vi "Base64.vi"(1 "Switch":enum16{"Base 64 Encode", "Base 64 Decode"}(ring), 2 "Input String":string, 4 "OutputFileStructure":bool) -> (6 "Output String":string)   [LabVIEW 2019, in "HTTP Server.lvlib"]
uses:
  HTTP Server.lvlib
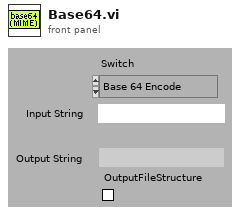
[diagram p1: front panel]
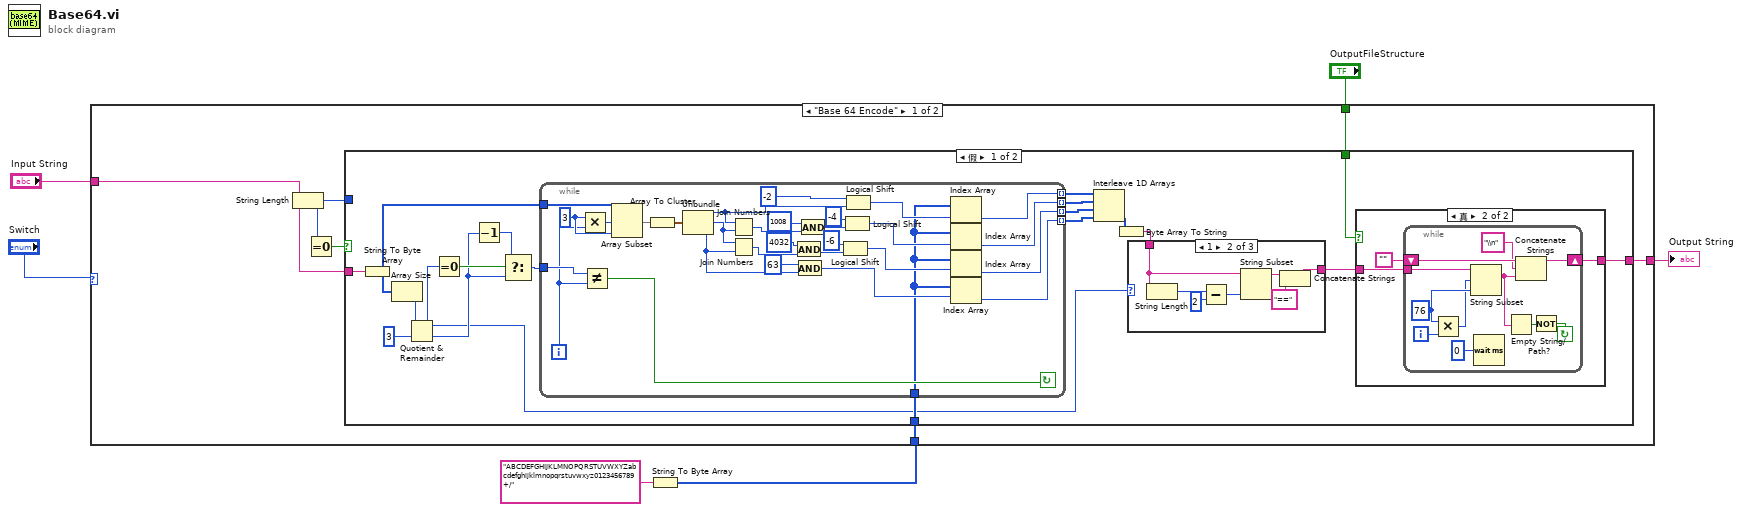
[diagram p0: block diagram]
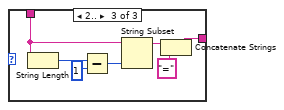
[diagram p3: hidden frame]
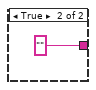
[diagram p5: hidden frame]
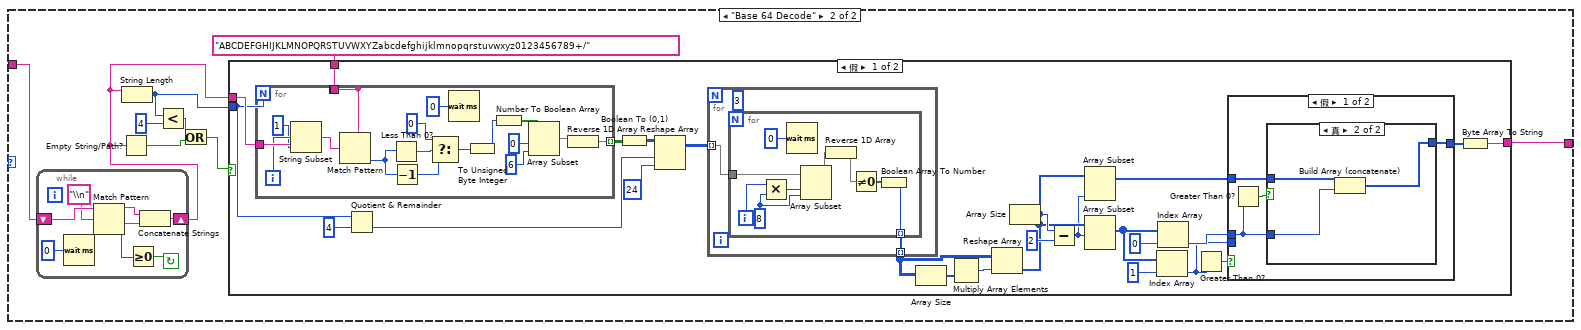
[diagram p6: hidden frame]
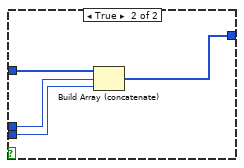
[diagram p8: hidden frame]
diagram:
  n1 = String To Byte Array(string="ABCDEFGHIJKLMNOPQRSTUVWXYZabcdefghijklmnopqrstuvwxyz0123456789+/") -> (unsigned byte array=w1:u8[])
  n2 = case shown="\"Base 64 Encode\"" "Switch" {
    tunnel: "Input String" -> [w12 w94]
    tunnel: "OutputFileStructure" -> [w11 _]
    tunnel: [w10 w98] -> w3
    tunnel: w1 -> [w7 _]
    frame "Base 64 Encode" {
      n3 = String Length(string=w12) -> (length=w8:i32)
      n4 = Equal To 0?(x=w8) -> (x = 0?=w9:bool)
      n5 = case shown="假" w9 {
        tunnel: [w31 ""] -> w10
        tunnel: w11 -> [w30 _]
        tunnel: w12 -> [w22 _]
        tunnel: w8 -> [_ _]
        tunnel: w7 -> [w24 _]
        frame False {
          n6 = String To Byte Array(string=w22) -> (unsigned byte array=w21:u8[])
          n7 = Array Size(array=w21) -> (size(s)=w25:i32)
          n8 = Quotient & Remainder(x=w25, y=3) -> (x-y*floor(x/y)=w14:i32, floor(x/y)=w28:i32)
          n9 = Equal To 0?(x=w14) -> (x = 0?=w29:bool)
          n10 = Decrement(x=w28) -> (x-1=w27:i32)
          n11 = Select(t=w27, s=w29, f=w28) -> (s? t:f=w23:i32)
          n12 = while {
            tunnel: [w32] -> w17 mode=indexing
            tunnel: [w33] -> w18 mode=indexing
            tunnel: [w34] -> w19 mode=indexing
            tunnel: [w35] -> w20 mode=indexing
            tunnel: w23 -> [w56]
            tunnel: w24 -> [w36]
            tunnel: w21 -> [w61]
            i -> [w55]
            stop <- w54 continue-if-true
            w59 = 3 ("x")
            n13 = Multiply(x=w59, y=w55) -> (x*y=w60:i32)
            n14 = Not Equal?(x=w56, y=w55) -> (x != y?=w54:bool)
            n15 = Array Subset(array=w61, index=w60, length=w59) -> (w57:u8[])
            n16 = Array To Cluster(array=w57) -> (cluster=w58:cluster{"[0]":u8, "[1]":u8, "[2]":u8})
            n17 = Unbundle(w58) -> ("[0]"=w43:u8, "[1]"=w48:u8, "[2]"=w42:u8)
            n18 = Join Numbers(hi=w43, lo=w48) -> ((hi.lo)=w52:u16)
            n19 = Join Numbers(hi=w48, lo=w42) -> ((hi.lo)=w47:u16)
            n20 = And(x=u16 4032, y=w47) -> (x .and. y?=w45:u16)
            n21 = And(x=u8 63, y=w42) -> (x .and. y?=w37:u8)
            n22 = And(x=u16 1008, y=w52) -> (x .and. y?=w50:u16)
            n23 = Logical Shift(y=i8 -6, x=w45) -> (x << y=w38:u16)
            n24 = Logical Shift(y=i8 -4, x=w50) -> (x << y=w39:u16)
            n25 = Logical Shift(y=i8 -2, x=w43) -> (x << y=w40:u8)
            n26 = Index Array(array=w36, index=w40) -> (element=w35:u8)
            n27 = Index Array(array=w36, index=w39) -> (element=w34:u8)
            n28 = Index Array(array=w36, index=w38) -> (element=w33:u8)
            n29 = Index Array(array=w36, index=w37) -> (element=w32:u8)
          }
          n30 = Interleave 1D Arrays(w20, w19, w18, w17) -> (w16:u8[])
          n31 = Byte Array To String(unsigned byte array=w16) -> (string=w15:string)
          n32 = case shown="1" w14 {
            tunnel: w15 -> [w62 w64 w71]
            tunnel: [w62 w63 w70] -> w13
            frame ..0 {
            }
            frame 1 {
              n33 = String Length(string=w64) -> (length=w68:i32)
              n34 = Subtract(x=w68, y=i16 2) -> (x-y=w67:i32)
              n35 = String Subset(string=w64, length (rest)=w67) -> (substring=w65:string)  [unwired: 1 out]
              n36 = Concatenate Strings(w65, "==") -> (w63:string)
            }
            frame 2.. {
              n37 = String Length(string=w71) -> (length=w75:i32)
              n38 = Subtract(x=w75, y=i16 1) -> (x-y=w74:i32)
              n39 = String Subset(string=w71, length (rest)=w74) -> (substring=w72:string)  [unwired: 1 out]
              n40 = Concatenate Strings(w72, "=") -> (w70:string)
            }
          }
          n41 = case shown="真" w30 {
            tunnel: [w77 w79] -> w31
            tunnel: w13 -> [w77 w78]
            frame False {
            }
            frame True {
              n42 = while {
                shift-left: "" -> [w88]
                shift-right: [w87] -> w79
                tunnel: w78 -> [w81]
                i -> [w91]
                stop <- w84 continue-if-true
                w90 = 76 ("length")
                n43 = Multiply(x=w90, y=w91) -> (x*y=w89:i32)
                n44 = String Subset(string=w81, offset (0)=w89, length (rest)=w90) -> (substring=w83:string)
                n45 = Wait (ms)(milliseconds to wait=u32 0) -> ()  [unwired: 1 out]
                n46 = Empty String/Path?(string/path=w83) -> (empty?=w85:bool)
                n47 = Concatenate Strings(w88, "\\n", w83) -> (w87:string)
                n48 = Not(x=w85) -> (.not. x?=w84:bool)
              }
            }
          }
        }
        frame True {
        }
      }
    }
    frame "Base 64 Decode" {
      n49 = while {
        shift-left: w94 -> [w105]
        shift-right: [w106] -> w93
        stop <- w107 continue-if-true
        n50 = Wait (ms)(milliseconds to wait=u32 0) -> ()  [unwired: 1 out]
        n51 = Match Pattern(string=w105, regular expression="\\n") -> (before substring=w108:string, after substring=w109:string, offset past match=w104:i32)  [unwired: 2 out]
        n52 = Greater Or Equal To 0?(x=w104) -> (x >= 0?=w107:bool)
        n53 = Concatenate Strings(w108, w109) -> (w106:string)
      }
      n54 = Empty String/Path?(string/path=w93) -> (empty?=w99:bool)
      n55 = String Length(string=w93) -> (length=w96:i32)
      n56 = Less?(x=w96, y=4) -> (x < y?=w100:bool)
      n57 = Or(x=w100, y=w99) -> (x .or. y?=w97:bool)
      n58 = case shown="假" w97 {
        tunnel: [w112 w176] -> w98
        tunnel: w93 -> [w134 w176]
        tunnel: w96 -> [w132 _]
        tunnel: "ABCDEFGHIJKLMNOPQRSTUVWXYZabcdefghijklmnopqrstuvwxyz0123456789+/" ("string") -> [w133 _]
        frame False {
          n59 = for {
            N: w132 -> [_]
            tunnel: w134 -> [w175]
            tunnel: [w171] -> _ mode=indexing
            tunnel: w133 -> [w171]
            tunnel: [w162] -> w128 mode=indexing
            i -> [w174]
            n60 = String Subset(string=w175, offset (0)=w174, length (rest)=1 ("length")) -> (substring=w172:string)
            n61 = Match Pattern(string=w171, regular expression=w172) -> (offset past match=w161:i32)  [unwired: 4 out]
            n62 = Less Than 0?(x=w161) -> (x < 0?=w169:bool)
            n63 = Decrement(x=w161) -> (x-1=w160:i32)
            n64 = Select(t=0, s=w169, f=w160) -> (s? t:f=w168:i32)
            n65 = Wait (ms)(milliseconds to wait=u32 0) -> ()  [unwired: 1 out]
            n66 = To Unsigned Byte Integer(number=w168) -> (unsigned 8bit integer=w167:u8)
            n67 = Number To Boolean Array(number=w167) -> (Boolean array=w166:bool[])
            n68 = Array Subset(array=w166, index=0, length=6) -> (w163:bool[])
            n69 = Reverse 1D Array(array=w163) -> (reversed array=w162:bool[])
          }
          n70 = Quotient & Remainder(x=w132, y=4) -> (floor(x/y)=w130:i32)  [unwired: 1 out]
          n71 = Boolean To (0,1)(Boolean=w128) -> (0, 1=w127:i16[][])
          n72 = Reshape Array(w127, w130, 24) -> (w126:i16[][])
          n73 = for {
            tunnel: w126 -> [w148] mode=indexing
            tunnel: [w147] -> w124 mode=indexing
            n74 = for {
              N: 3 -> [_]
              tunnel: w148 -> [w157]
              tunnel: [w151] -> w147 mode=indexing
              i -> [w158]
              w155 = 8 ("y")
              n75 = Multiply(x=w158, y=w155) -> (x*y=w156:i32)
              n76 = Wait (ms)(milliseconds to wait=u32 0) -> ()  [unwired: 1 out]
              n77 = Array Subset(array=w157, index=w156, length=w155) -> (w154:i16[])
              n78 = Reverse 1D Array(array=w154) -> (reversed array=w153:i16[])
              n79 = Not Equal To 0?(x=w153) -> (x != 0?=w152:bool[])
              n80 = Boolean Array To Number(Boolean array=w152) -> (number=w151:u32)
            }
          }
          n81 = Array Size(array=w124) -> (size(s)=w125:i32[])
          n82 = Multiply Array Elements(1:w125) -> (0:w123:i32)
          n83 = Reshape Array(w124, w123) -> (w120:u32[])
          n84 = Array Size(array=w120) -> (size(s)=w122:i32)
          n85 = Subtract(x=w122, y=2) -> (x-y=w119:i32)
          n86 = Array Subset(array=w120, length=w119) -> (w114:u32[])  [unwired: 1 in]
          n87 = Array Subset(array=w120, index=w119) -> (w116:u32[])  [unwired: 1 in]
          n88 = Index Array(array=w116, index=1) -> (element=w113:u32)
          n89 = Index Array(array=w116, index=0) -> (element=w118:u32)
          n90 = Greater Than 0?(x=w113) -> (x > 0?=w117:bool)
          n91 = case shown="假" w117 {
            tunnel: w118 -> [w136 w145]
            tunnel: w114 -> [w137 w146]
            tunnel: w113 -> [_ w144]
            tunnel: [w135 w143] -> w111
            frame False {
              n92 = Greater Than 0?(x=w136) -> (x > 0?=w138:bool)
              n93 = case shown="真" w138 {
                tunnel: w137 -> [w139 w142]
                tunnel: w136 -> [_ w141]
                tunnel: [w139 w140] -> w135
                frame False {
                }
                frame True {
                  n94 = Build Array (concatenate)(w142, w141) -> (w140:u32[])
                }
              }
            }
            frame True {
              n95 = Build Array (concatenate)(w146, w145, w144) -> (w143:u32[])
            }
          }
          n96 = Byte Array To String(unsigned byte array=w111) -> (string=w112:string)
        }
        frame True {
        }
      }
    }
  }
  "Output String" <- w3
